vi "sv_Frequency Weighting Characteristic.vi"(1 "spectrum type":enum16{"Power", "Amplitude"}(ring), 2 "dB On (T)":bool=TRUE, 3 "frequency [Hz]":dbl=1000.0 min=0.0 format="%.2f", 4 "weighting filter":T1 items=["Linear", "A-weighting", "B-weighting", "C-weighting", "ITU-R 468-4", "Dolby", "CCITT", "C-message", "Wb", "Wc", "Wd", "We", "Wf", "Wh", "Wj", "Wk", "Wm", "AES17 20 kHz lowpass", "AES17 40 kHz lowpass", "AES17 20 kHz highpass", "AES17 40 kHz highpass"]) -> (0 "relative response level":dbl format="%.2f")   [LabVIEW 2017]
uses:
  <vilib>/addons/_NISVFA/_Shared subVIs/Controls/svc_Weighting Filter Text Ring.ctl
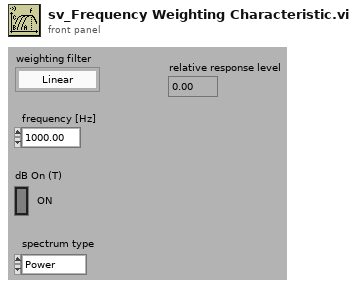
[diagram p1: front panel]
types:
  T1 = typedef "svc_Weighting Filter Text Ring.ctl" = u16
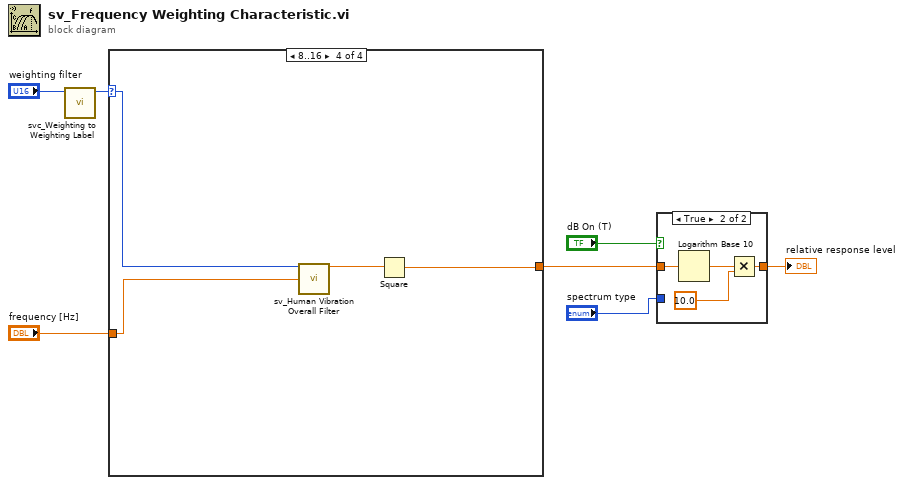
[diagram p0: block diagram]
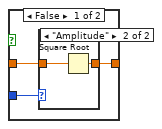
[diagram p2: hidden frame]
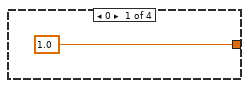
[diagram p4: hidden frame]
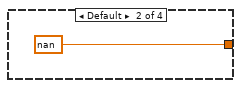
[diagram p5: hidden frame]
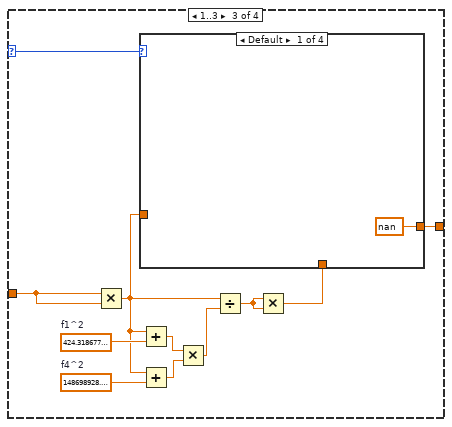
[diagram p6: hidden frame]
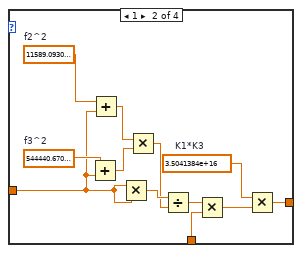
[diagram p7: hidden frame]
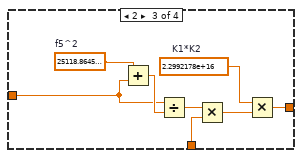
[diagram p8: hidden frame]
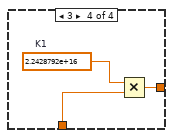
[diagram p9: hidden frame]
diagram:
  n1 = call <vilib>:"svc_Weighting to Weighting Label.vi"("weighting filter"="weighting filter") -> ("weighting enum"=w3:T1)  [unwired: 9 in, 1 out]
  n2 = case shown="8..16" w3 {
    selector: w3 -> [_ _ w11 w48]
    tunnel: [1.0 nan w12 w45] -> w1
    tunnel: "frequency [Hz]" -> [_ _ w10 w47]
    frame 0 {
    }
    frame Default {
    }
    frame 1..3 {
      w15 = 148698928.24308902  # f4^2
      w16 = 424.31867740600904  # f1^2
      n3 = Multiply(x=w10, y=w10) -> (x*y=w13:dbl)
      n4 = Add(x=w13, y=w16) -> (x+y=w18:dbl)
      n5 = Add(x=w13, y=w15) -> (x+y=w19:dbl)
      n6 = Multiply(x=w18, y=w19) -> (x*y=w17:dbl)
      n7 = Divide(x=w13, y=w17) -> (x/y=w20:dbl)
      n8 = Multiply(x=w20, y=w20) -> (x*y=w14:dbl)
      n9 = case shown="Default" w11 {
        tunnel: [nan w33 w41 w44] -> w12
        tunnel: w14 -> [_ w31 w38 w43]
        tunnel: w13 -> [_ w22 w36 _]
        frame Default {
        }
        frame 1 {
          w23 = 544440.6704605728  # f3^2
          w24 = 11589.0930520225  # f2^2
          w27 = 3.5041384e+16  # K1*K3
          n10 = Add(x=w23, y=w22) -> (x+y=w26:dbl)
          n11 = Add(x=w24, y=w22) -> (x+y=w29:dbl)
          n12 = Multiply(x=w22, y=w22) -> (x*y=w28:dbl)
          n13 = Multiply(x=w29, y=w26) -> (x*y=w25:dbl)
          n14 = Divide(x=w28, y=w25) -> (x/y=w32:dbl)
          n15 = Multiply(x=w32, y=w31) -> (x*y=w30:dbl)
          n16 = Multiply(x=w27, y=w30) -> (x*y=w33:dbl)
        }
        frame 2 {
          w35 = 25118.8645540624  # f5^2
          w34 = 2.2992178e+16  # K1*K2
          n17 = Add(x=w35, y=w36) -> (x+y=w40:dbl)
          n18 = Divide(x=w36, y=w40) -> (x/y=w39:dbl)
          n19 = Multiply(x=w39, y=w38) -> (x*y=w37:dbl)
          n20 = Multiply(x=w34, y=w37) -> (x*y=w41:dbl)
        }
        frame 3 {
          w42 = 2.2428792e+16  # K1
          n21 = Multiply(x=w42, y=w43) -> (x*y=w44:dbl)
        }
      }
    }
    frame 8..16 {
      n22 = call <vilib>:"sv_Human Vibration Overall Filter.vi"("weighting enum"=w48, "f"=w47) -> ("|Hh(s)*Hl(s)*Ht(s)*Hs(s)|"=w46:dbl)  [unwired: 11 in, 2 out]
      n23 = Square(x=w46) -> (x^2=w45:dbl)
    }
  }
  n24 = case shown="True" "dB On (T)" {
    tunnel: w1 -> [w50 w57]
    tunnel: [w51 w56] -> w6
    tunnel: "spectrum type" -> [w49 _]
    frame False {
      n25 = case shown="\"Amplitude\"" w49 {
        tunnel: [w52 w54] -> w51
        tunnel: w50 -> [w52 w53]
        frame "Power", Default {
        }
        frame "Amplitude" {
          n26 = Square Root(x=w53) -> (sqrt(x)=w54:dbl)
        }
      }
    }
    frame True {
      n27 = Logarithm Base 10(1:w57) -> (0:w58:dbl)
      n28 = Multiply(x=w58, y=10.0) -> (x*y=w56:dbl)
    }
  }
  "relative response level" <- w6
